vi "Autotuning PID PWM.vi"() -> ()   [LabVIEW 2015]
doc: "This example demonstrates how to use the PID Design function to obtain PID parameters based on measured process."
uses:
  <vilib>/addons/control/pid/pid.llb/PID Advanced (DBL).vi
  <vilib>/addons/control/pid/autopid.llb/PID Autotuning Design (Ziegler-Nichols).vi
  <vilib>/addons/control/pid/autopid.llb/PID Autotuning Design (Cohen-Coon).vi
  <vilib>/addons/control/pid/autopid.llb/PID Autotuning Design (Chien-Hrones-Reswick).vi
  <vilib>/addons/control/pid/autopid.llb/PID Autotuning Design (Internal Model Control).vi
  <vilib>/addons/control/pid/NI_PID_autopid.lvlib
  <vilib>/addons/control/pid/NI_PID_pid.lvlib
  <vilib>/ptbypt/NI_PtbyPt.lvlib
panel:
  in  "Excitation":dbl=0.5 format="%.2f"
  in  "Type of controller":u16(ring)=2 items=["P", "PI", "PID"]
  in  "Control":T1(tab)
  in  "Ziegler-Nichols speed":u16(ring) items=["Fast", "Normal", "Slow"]
  in  "Tuning specifications":u16(ring) items=["Regulator - 0 %", "Regulator -  20%", "Servo - 0%", "Servo - 20%"]
  in  "Multiplicative factor":dbl(slide)=1.0 scale=0.01..100.0
  in  "Tab Control":T2(tab)
  in  "Instructions":string="Overview: This example demonstrates how to use the PID Autotuning Design to obtain PID parameters based on setpoint and process variable collected in another loop.\nInstructions:\n1. Run the VI and wait until the process variable (PV) reaches near setpoint (SP).\n2.  In the PID Autotuning Design section, select the type of algorithm, type of controller and excitation amplitude for the 'open loop step response'. Then, click Autotune to start the process. Select the Identified Plant Parameter tab and see the results from the identification.\n3.  When the tuned PID gains do not change anymore, the identification is done and you have the option to accept by clicking Accept gain, which will transfer the new gain to PID Gains.\n4. Click the Autotune button again to go back to the automatic control state. You can try different options and repeat this process.\n5. Click Stop to stop the VI.\n"
  out "Identified Plant Parameters":T3={"Plant Gain (K)"=1.7609511324977591, "Time Constant (T)"=1.9621978490901302, "Dead Time (L)"=0.22467425343567116}
  out "Control Output":dbl[](graph)
  out "Measurement":dbl[](graph)
  out "Stimulus operating point":dbl=20.314221540357543
  out "Response operating point":dbl=51.08345461694337
  in  "Automatic":bool=TRUE
  in  "Reinitialize":bool
  out "MV":dbl(graph)=20.39115328927357
  in  "Accept gain":bool
  out "Tuned PID gains":T4={"proportional gain (Kc)"=1.9838195929127882, "integral time (Ti, min)"=0.01995856284686879, "derivative time (Td, min)"=0.0} {"derivative time (Td, min)" format="%#.6g"; "integral time (Ti, min)" format="%#.6g"; "proportional gain (Kc)" format="%#.6g"}
  in  "Autotune":bool
  in  "SP:":dbl(slide)=50.98039215686275 min=0.0 max=0.0 scale=0.0..100.0
  in  "MV:":dbl(slide)=20.39115328927357 scale=-100.0..100.0
  out "PV:":dbl(slide)=50.98160323470328 scale=0.0..100.0
  in  "PID Gains":T4={"proportional gain (Kc)"=2.5, "integral time (Ti, min)"=0.02, "derivative time (Td, min)"=0.0} {"derivative time (Td, min)" format="%#.6g"; "integral time (Ti, min)" format="%#.6g"; "proportional gain (Kc)" format="%#.6g"}
  in  "Sampling Time dt (s)":dbl=0.05 min=0.001 step=0.01 format="%#.3p"
  in  "Stop":bool
  out "SP and PV":cluster{"initial PV":dbl, "SP1:":dbl}(graph)={"initial PV"=50.98160323470328, "SP1:"=50.98039215686275}
  # "Proportional-Integral-Derivative (PID) Controller"
  # "PID Autotuning Design"
  # "No additional parameters"
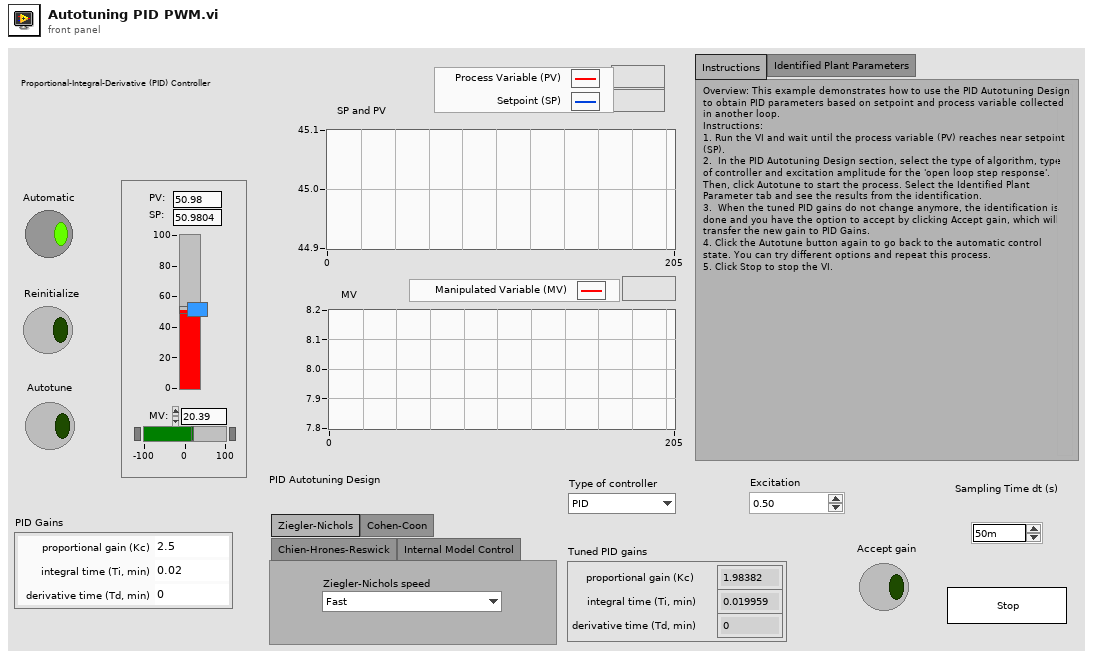
[diagram p1: front panel]
types:
  T1 = enum32{"Ziegler-Nichols", "Cohen-Coon", "Chien-Hrones-Reswick", "Internal Model Control"}
  T2 = enum32{"Instructions", "Identified Plant Parameters"}
  T3 = cluster{"Plant Gain (K)":dbl, "Time Constant (T)":dbl, "Dead Time (L)":dbl}
  T4 = cluster{"proportional gain (Kc)":dbl, "integral time (Ti, min)":dbl, "derivative time (Td, min)":dbl}
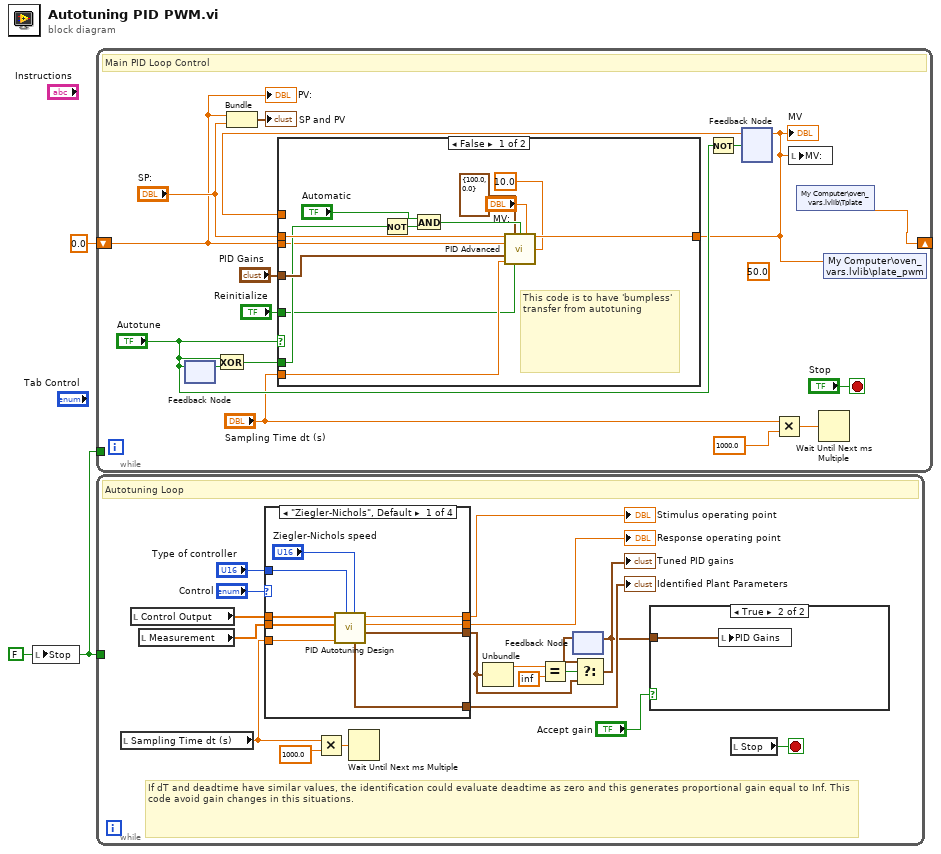
[diagram p0: block diagram]
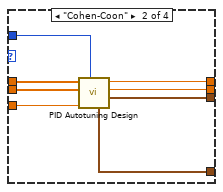
[diagram p2: hidden frame]
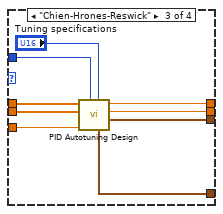
[diagram p3: hidden frame]
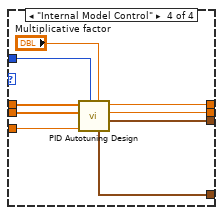
[diagram p4: hidden frame]
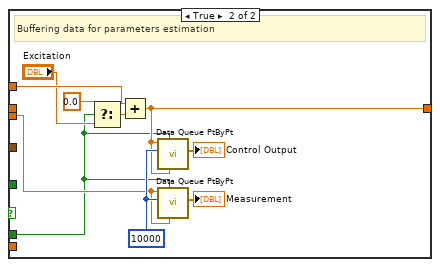
[diagram p6: hidden frame]
diagram:
  w1 = FALSE ("Stop")
  n1 = local write "Stop"(w1) -> ()
  n2 = while {
    shift-left: 0.0 ("Plant Output") -> [w11]
    shift-right: [w4] -> _
    tunnel: w1 -> [_]
    stop <- "Stop" stop-if-true
    (unwired) 50.0 ("y")
    # "Main PID Loop Control"
    n3 = feedback #1() -> (w13:bool)  [unwired: 1 in]
    n4 = feedback-in #1("Autotune") -> ()
    n5 = Exclusive Or(1:w13, 2:"Autotune") -> (0:w12:bool)
    n6 = Bundle("Plant Output"=w11, "SP:"="SP:") -> (→"SP and PV":cluster{"Plant Output":dbl, "SP:":dbl})  [unwired: 1 in]
    n7 = Not(x="Autotune") -> (.not. x?=w8:bool)
    n8 = feedback #2() -> (w10:dbl)  [unwired: 1 in]
    n9 = case shown="False" "Autotune" {
      tunnel: "Sampling Time dt (s)" -> [w31 _]
      tunnel: [w29 w34] -> w3
      tunnel: w11 -> [w26 w33]
      tunnel: "SP:" -> [w28 _]
      tunnel: "PID Gains" -> [w30 _]
      tunnel: "Reinitialize" -> [w24 _]
      tunnel: w12 -> [w27 w32]
      tunnel: w10 -> [_ w38]
      frame False {
        # "This code is to have 'bumpless' transfer from autotuning"
        n10 = Not(x=w27) -> (.not. x?=w23:bool)
        n11 = And(x="Automatic", y=w23) -> (x .and. y?=w25:bool)
        n12 = call-poly <vilib>:"PID Advanced.vi"("setpoint"=w28, "output range"=cluster{"output high":dbl, "output low":dbl} {"output high"=100.0, "output low"=0.0}, "auto? (T)"=w25, "manual control"="MV:", "process variable"=w26, "alpha"=10.0, "PID gains"=w30, "dt (s)"=w31, "reinitialize? (F)"=w24) -> ("output"=w29:dbl)  [unwired: 5 in, 1 out]
      }
      frame True {
        w41 = 10000 ("sample length")
        # "Buffering data for parameters estimation"
        n13 = Select(t=0.0, s=w32, f="Excitation") -> (s? t:f=w39:dbl)
        n14 = Add(x=w38, y=w39) -> (x+y=w34:dbl)
        n15 = call <vilib>:"Data Queue PtByPt.vi"("initial queue element"=w34, "initialize"=w32, "sample length"=w41, "input data point"=w34) -> ("Current Queue"=→"Control Output":dbl[])  [unwired: 3 in, 4 out]
        n16 = call <vilib>:"Data Queue PtByPt.vi"("initial queue element"=w33, "initialize"=w32, "sample length"=w41, "input data point"=w33) -> ("Current Queue"=→"Measurement":dbl[])  [unwired: 3 in, 4 out]
      }
    }
    "MV" <- w3
    n17 = feedback-in #2(w3, w8) -> ()
    n18 = Multiply(x="Sampling Time dt (s)", y=1000.0) -> (x*y=w6:dbl)
    n19 = local write "MV:"(w3) -> ()
    n20 = shared-variable "My Computer\\oven_vars.lvlib\\Tplate"() -> (w4:dbl)  [unwired: 1 in, 1 out]
    n21 = Wait Until Next ms Multiple(millisecond multiple=w6) -> ()  [unwired: 1 out]
    n22 = shared-variable "My Computer\\oven_vars.lvlib\\plate_pwm"(w3) -> ()  [unwired: 1 in, 1 out]
    "PV:" <- w11
  }
  n23 = while {
    tunnel: w1 -> [_]
    stop <- w54 stop-if-true
    # "If dT and deadtime have similar values, the identification could evaluate deadtime as zero and this generates proportional gain equal to Inf. This code avoid gain changes in this situations."
    # "Autotuning Loop"
    n24 = local read "Sampling Time dt (s)"() -> (w55:dbl)
    n25 = local read "Control Output"() -> (w59:dbl[])
    n26 = local read "Measurement"() -> (w58:dbl[])
    n27 = case shown="\"Ziegler-Nichols\", Default" "Control" {
      tunnel: w59 -> [w68 w76 w85 w94]
      tunnel: w58 -> [w67 w75 w84 w93]
      tunnel: [w66 w74 w83 w92] -> w57
      tunnel: [w65 w73 w82 w91] -> w56
      tunnel: w55 -> [w64 w72 w81 w90]
      tunnel: [w63 w71 w80 w89] -> w52
      tunnel: [w62 w70 w79 w88] -> w43
      tunnel: "Type of controller" -> [w61 w69 w78 w87]
      frame "Ziegler-Nichols", Default {
        n28 = call-poly <vilib>:"PID Autotuning Design.vi"("Ziegler-Nichols Speed"="Ziegler-Nichols speed", "Type of Controller"=w61, "dt (s)"=w64, "Response signal"=w67, "Stimulus signal"=w68) -> ("PID gains"=w62:T4, "response operating point"=w65:dbl, "stimulus operating point"=w66:dbl, "Plant Parameters"=w63:T3)  [unwired: 3 in]
      }
      frame "Cohen-Coon" {
        n29 = call-poly <vilib>:"PID Autotuning Design.vi"("Type of Controller"=w69, "dt (s)"=w72, "Response signal"=w75, "Stimulus signal"=w76) -> ("PID gains"=w70:T4, "response offset"=w73:dbl, "stimulus offset"=w74:dbl, "Plant Parameters"=w71:T3)  [unwired: 4 in]
      }
      frame "Chien-Hrones-Reswick" {
        n30 = call-poly <vilib>:"PID Autotuning Design.vi"("Tuning specifications"="Tuning specifications", "Type of Controller"=w78, "dt (s)"=w81, "Response signal"=w84, "Stimulus signal"=w85) -> ("PID gains"=w79:T4, "response offset"=w82:dbl, "stimulus offset"=w83:dbl, "Plant Parameters"=w80:T3)  [unwired: 3 in]
      }
      frame "Internal Model Control" {
        n31 = call-poly <vilib>:"PID Autotuning Design.vi"("Desired Time Constant (tau_c)"="Multiplicative factor", "Type of Controller"=w87, "dt (s)"=w90, "Response signal"=w93, "Stimulus signal"=w94) -> ("PID gains"=w88:T4, "response offset"=w91:dbl, "stimulus offset"=w92:dbl, "Plant Parameters"=w89:T3)  [unwired: 3 in]
      }
    }
    "Stimulus operating point" <- w57
    "Response operating point" <- w56
    "Identified Plant Parameters" <- w52
    n32 = Multiply(x=w55, y=1000.0) -> (x*y=w51:dbl)
    n33 = Wait Until Next ms Multiple(millisecond multiple=w51) -> ()  [unwired: 1 out]
    n34 = Unbundle(w43) -> ("proportional gain (Kc)"=w46:dbl)  [unwired: 2 out]
    n35 = Equal?(x=w46, y=inf) -> (x = y?=w45:bool)
    n36 = feedback #3() -> (w44:T4)  [unwired: 1 in]
    n37 = Select(t=w44, s=w45, f=w43) -> (s? t:f=w42:T4)
    "Tuned PID gains" <- w42
    n38 = feedback-in #3(w42) -> ()
    n39 = case shown="True" "Accept gain" {
      tunnel: w42 -> [_ w95]
      frame False {
      }
      frame True {
        n40 = local write "PID Gains"(w95) -> ()
      }
    }
    n41 = local read "Stop"() -> (w54:bool)
  }
